vi "Post-Build.vi"(5 "Files Generated by Build":path[](array[path]), 6 "Top Level/Always Included VIs":path[](array[path]), 7 "Destination Path":path, 8 "error in (no error)":errorcluster, 9 "Target Name":string, 10 "Build Specification Name":string, 11 "Project Path":path) -> (0 "error out":errorcluster)   [LabVIEW 2015]
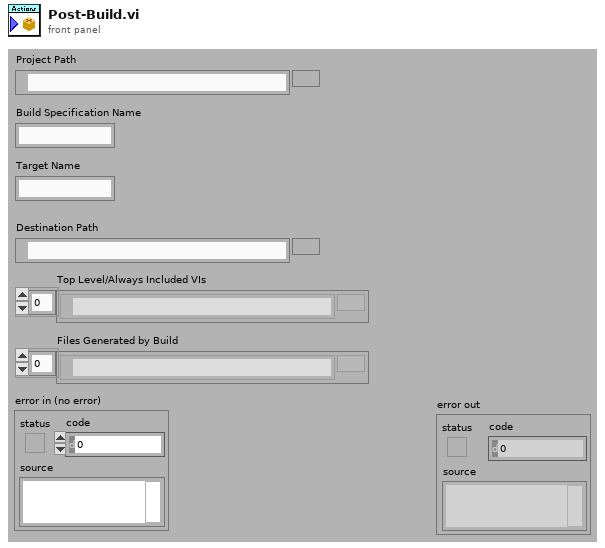
[diagram p1: front panel]
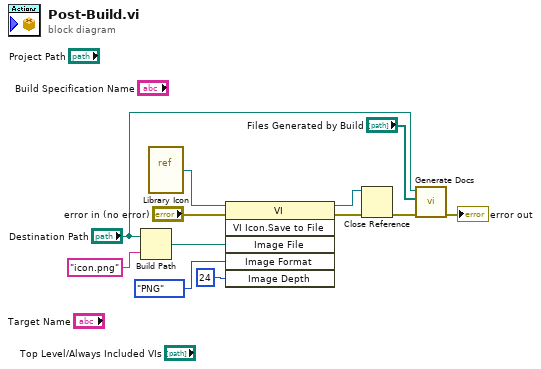
[diagram p0: block diagram]
diagram:
  n1 = Build Path(base path="Destination Path", name or relative path="icon.png") -> (appended path=w8:path)
  n2 = vi-ref "Library Icon.vi"() -> (w12:refnum<vi>)
  n3 = invoke class="VI" method="VI Icon.Save to File"(reference=w12, error in="error in (no error)", "Image File"=w8, "Image Format"=enum32{"PNG", "JPEG", "GIF", "BMP"}."PNG", "Image Depth"=24) -> (reference out=w5:refnum<vi>, error out=w6:errorcluster)  [unwired: 1 in, 4 out]
  n4 = Close Reference(reference=w5, error in (no error)=w6) -> (error out=w4:errorcluster)
  n5 = call "Generate Docs.vi"("error in (no error)"=w4, "Files Generated by Build"="Files Generated by Build", "Destination Path"="Destination Path") -> ("error out"=→"error out":errorcluster)  [unwired: 8 in]
